vi "_051.vi"() -> ()   [LabVIEW 2024]
panel:
  out "Count Down":i32
  out "Count Up":i32
  in  "stop":bool
  in  "Counter":bool
  # "Count up & Count down :"
  # "( for each click )"
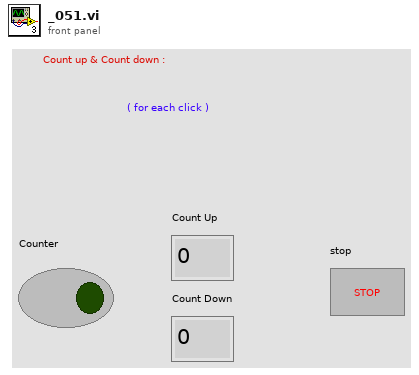
[diagram p1: front panel]
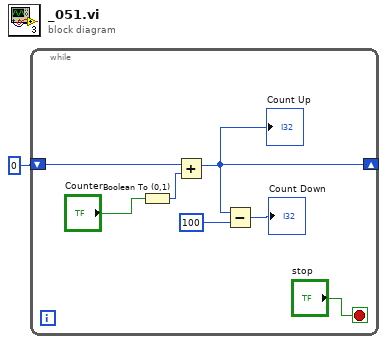
[diagram p0: block diagram]
diagram:
  n1 = while {
    shift-right: [w4] -> _
    shift-left: 0 -> [w7]
    stop <- "stop" stop-if-true
    n2 = Boolean To (0,1)(Boolean="Counter") -> (0, 1=w5:i16)
    n3 = Add(x=w7, y=w5) -> (x+y=w4:i32)
    "Count Up" <- w4
    n4 = Subtract(x=w4, y=100) -> (x-y=→"Count Down":i32)
  }
